vi "CheckOut.vi"(0 "Student List In":string[][](array[string]), 1 "Student ID":i32, 2 "date/time string":string, 3 "Checkin Flag":T1, 4 "Check Out":T1, 5 "Total Seconds":T1) -> (14 "Student List Out":string[][](array[string]), 16 "Total Elapsed Time":i32)   [LabVIEW 2013]
doc: "Writes a row of data to the row of 2D table of data. Each \nrow corresponds to a unique student. When a student checks out,\n\nCheckin Flag = FALSE\nCheck Out (Timestamp) = Current Time Stamp\n\nHours, Minutes, and Seconds are set to the value of the current time stamp, and \nsent to Check Out Logic.VI and used to calculate the time differential between \nCheck In and Check Out"
uses:
  Controls/SpreadsheetColumns.ctl
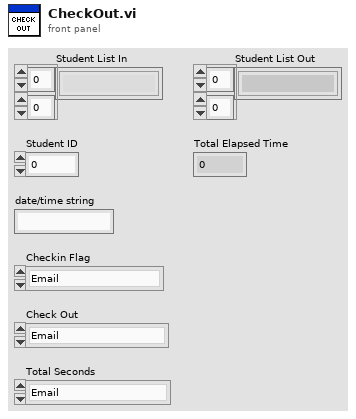
[diagram p1: front panel]
types:
  T1 = typedef "SpreadsheetColumns.ctl" = enum16{"Email", "CheckIn", "CheckOut", "Checkin Flag", "Hours", "Minutes", "Seconds", "Total Seconds", "Cat Points"}
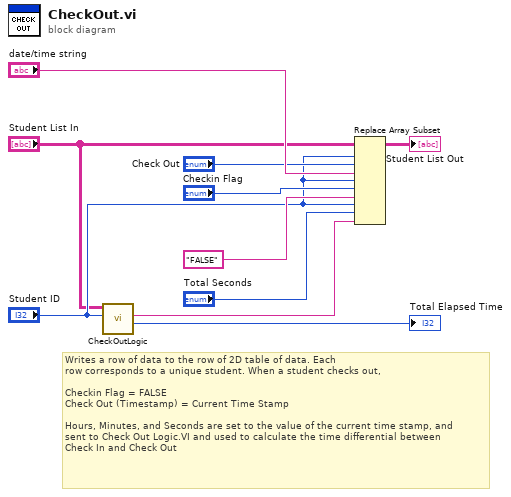
[diagram p0: block diagram]
diagram:
  # "Writes a row of data to the row of 2D table of data. Each \nrow corresponds to a unique student. When a student checks out,\n\nCheckin Flag = FALSE\nCheck Out (Timestamp) = Current Time Stamp\n\nHours, Minutes, and Seconds are set to the value of the current time stamp, and \nsent to Check Out Logic.VI and used to calculate the time differential between \nCheck In and Check Out"
  n1 = call "CheckOutLogic.vi"("Student ID"="Student ID", "Student List In"="Student List In") -> ("Total Elapsed Time"=→"Total Elapsed Time":i32, "Total Seconds Out"=w6:string)  [unwired: 7 in, 1 out]
  n2 = Replace Array Subset(array="Student List In", new element #1="date/time string", index (row) #1="Student ID", index (col) #1="Check Out", new element #2="FALSE" ("new element/subarray"), index (row) #2="Student ID", index (col) #2="Checkin Flag", new element #3=w6, index (row) #3="Student ID", index (col) #3="Total Seconds") -> (→"Student List Out":string[][])
